vi "CRYHarmonics list add item.vi"(9 "Checkoffs":bool[](array[boolean]), 10 "Items":string[](array[string]), 11 "Candidate item":string) -> (0 "Cancel operation":bool, 1 "Checkoffs out":bool[](array[boolean]), 2 "Items out":string[](array[string]))   [LabVIEW 2013]
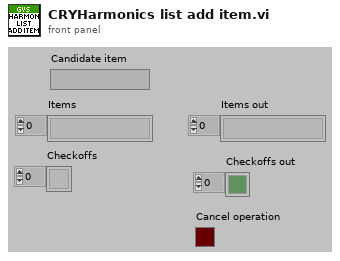
[diagram p1: front panel]
types:
  T1 = cluster{dbl, dbl, "String":string, "Boolean":bool}
  T2 = cluster{dbl, dbl, "Candidate item":string, "Boolean":bool}[]
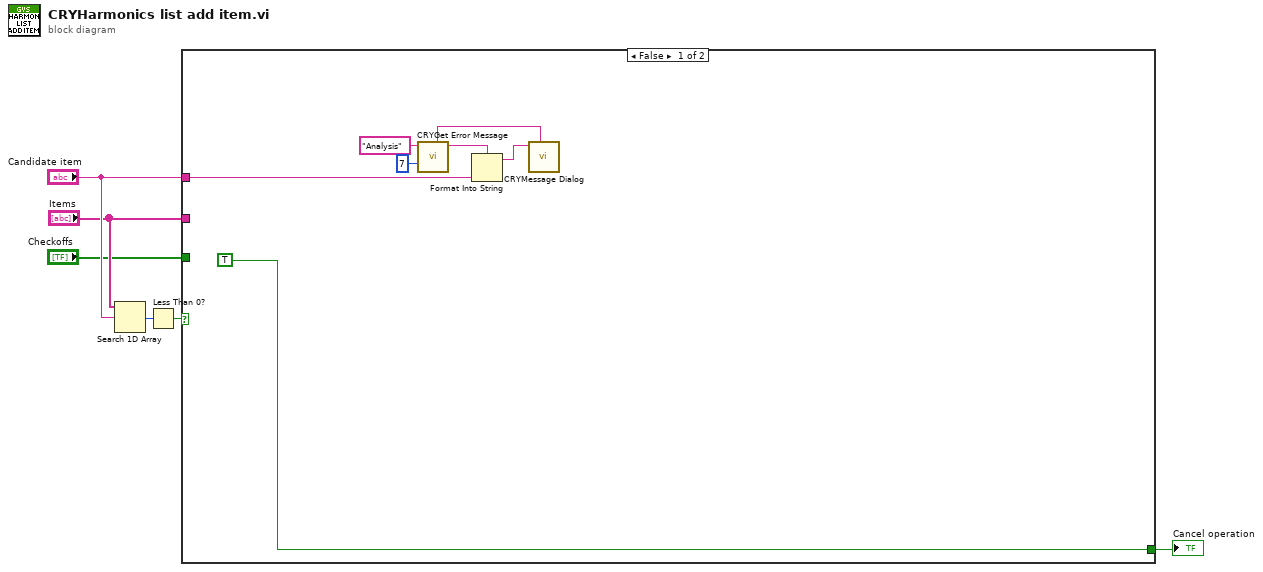
[diagram p0: block diagram]
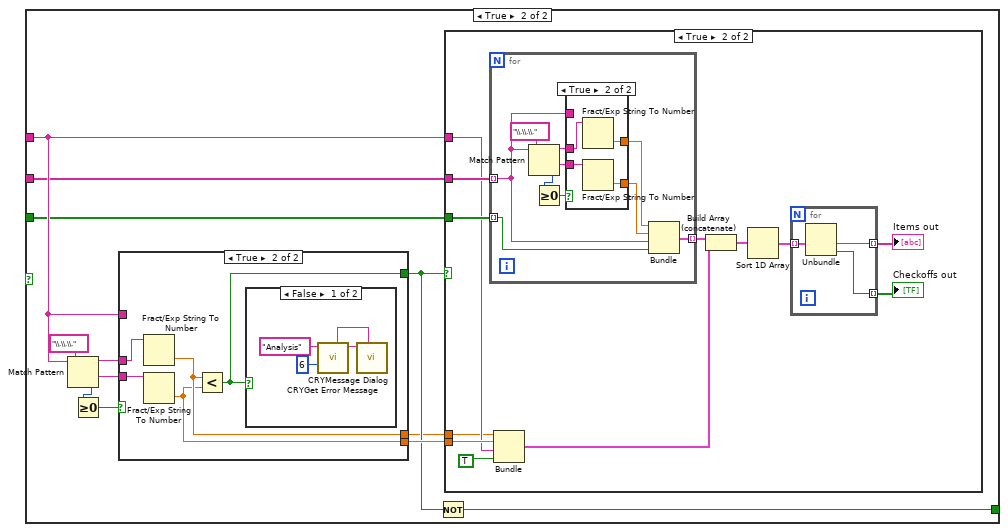
[diagram p2: hidden frame]
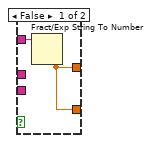
[diagram p4: hidden frame]
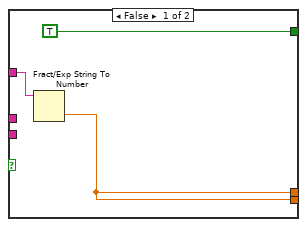
[diagram p5: hidden frame]
diagram:
  n1 = Search 1D Array(1D array="Items", element="Candidate item") -> (index of element=w6:i32)  [unwired: 1 out]
  n2 = Less Than 0?(x=w6) -> (x < 0?=w5:bool)
  n3 = case shown="False" w5 {
    tunnel: "Candidate item" -> [w8 w22]
    tunnel: "Items" -> [_ w21]
    tunnel: "Checkoffs" -> [_ w20]
    tunnel: [TRUE w17] -> w1
    frame False {
      n4 = call "CRYGet Error Message.vi"("Error No"=7, "Kind"="Analysis") -> ("Message"=w9:string, "Window Title"=w12:string)  [unwired: 4 in, 4 out]
      n5 = Format Into String(format string=w9, w8) -> (resulting string=w7:string)  [unwired: 2 in, 1 out]
      n6 = call "CRYMessage Dialog.vi"("Window Title"=w12, "Message Content"=w7) -> ()  [unwired: 8 in, 2 out]
    }
    frame True {
      n7 = Match Pattern(string=w22, regular expression="\\.\\.\\.") -> (before substring=w16:string, after substring=w15:string, offset past match=w24:i32)  [unwired: 2 out]
      n8 = Greater Or Equal To 0?(x=w24) -> (x >= 0?=w23:bool)
      n9 = case shown="True" w23 {
        tunnel: w22 -> [w59 _]
        tunnel: [w57 w60] -> w19
        tunnel: [TRUE w64] -> w18
        tunnel: w16 -> [_ w63]
        tunnel: w15 -> [_ w62]
        tunnel: [w57 w61] -> w14
        frame False {
          n10 = Fract/Exp String To Number(string=w59) -> (number=w57:dbl)  [unwired: 4 out]
        }
        frame True {
          n11 = Fract/Exp String To Number(string=w63) -> (number=w61:dbl)  [unwired: 4 out]
          n12 = Fract/Exp String To Number(string=w62) -> (number=w60:dbl)  [unwired: 4 out]
          n13 = Less?(x=w61, y=w60) -> (x < y?=w64:bool)
          n14 = case shown="False" w64 {
            frame False {
              n15 = call "CRYGet Error Message.vi"("Error No"=6, "Kind"="Analysis") -> ("Message"=w67:string, "Window Title"=w68:string)  [unwired: 4 in, 4 out]
              n16 = call "CRYMessage Dialog.vi"("Window Title"=w68, "Message Content"=w67) -> ()  [unwired: 8 in, 2 out]
            }
            frame True {
            }
          }
        }
      }
      n17 = Not(x=w18) -> (.not. x?=w17:bool)
      n18 = case shown="True" w18 {
        tunnel: w22 -> [_ w33]
        tunnel: w21 -> [_ w35]
        tunnel: w20 -> [_ w34]
        tunnel: w19 -> [_ w37]
        tunnel: w14 -> [_ w26]
        frame False {
        }
        frame True {
          n19 = for {
            tunnel: w35 -> [w47] mode=indexing
            tunnel: w34 -> [w46] mode=indexing
            tunnel: [w45] -> w32 mode=indexing
            n20 = Match Pattern(string=w47, regular expression="\\.\\.\\.") -> (before substring=w44:string, after substring=w43:string, offset past match=w50:i32)  [unwired: 2 out]
            n21 = Greater Or Equal To 0?(x=w50) -> (x >= 0?=w49:bool)
            n22 = case shown="True" w49 {
              tunnel: w47 -> [w52 _]
              tunnel: [w51 w56] -> w42
              tunnel: w44 -> [_ w55]
              tunnel: w43 -> [_ w54]
              tunnel: [w51 w53] -> w41
              frame False {
                n23 = Fract/Exp String To Number(string=w52) -> (number=w51:dbl)  [unwired: 4 out]
              }
              frame True {
                n24 = Fract/Exp String To Number(string=w55) -> (number=w56:dbl)  [unwired: 4 out]
                n25 = Fract/Exp String To Number(string=w54) -> (number=w53:dbl)  [unwired: 4 out]
              }
            }
            n26 = Bundle(w42, w41, "String"=w47, "Boolean"=w46) -> (w45:T1)  [unwired: 1 out]
          }
          n27 = Bundle(w26, w37, "Candidate item"=w33, TRUE) -> (w31:cluster{dbl, dbl, "Candidate item":string, bool})  [unwired: 1 out]
          n28 = Build Array (concatenate)(w32, w31) -> (w30:T2)
          n29 = Sort 1D Array(array=w30) -> (sorted array=w29:T2)
          n30 = for {
            tunnel: w29 -> [w40] mode=indexing
            tunnel: [w39] -> w28 mode=indexing
            tunnel: [w38] -> w27 mode=indexing
            n31 = Unbundle(w40) -> ("Candidate item"=w39:string, "Boolean"=w38:bool)  [unwired: 2 out]
          }
          "Items out" <- w28
          "Checkoffs out" <- w27
        }
      }
    }
  }
  "Cancel operation" <- w1
